vi "Pressure Write Array.vi"(8 "error in":errorcluster, 10 "Pressure AV":dbl[](array[numeric]), 11 "Chiller in":refnum<class "Chiller.lvclass">) -> (0 "error out":errorcluster, 3 "Chiller out":refnum<class "Chiller.lvclass">)   [LabVIEW 2023, in "Chiller.lvclass"]
uses:
  Chiller.lvclass
  Chiller.lvclass/Chiller.ctl
  Low Level Capabilities/Pressure/Pressure Actual Value/Pressure Actual Value.lvclass
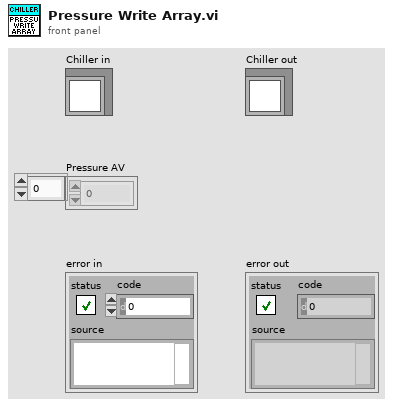
[diagram p1: front panel]
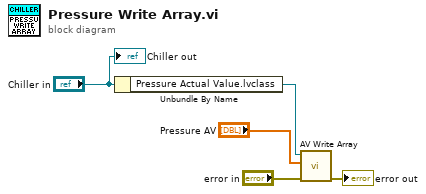
[diagram p0: block diagram]
diagram:
  n1 = Unbundle By Name("Chiller in") -> ("Pressure Actual Value.lvclass"=w5:refnum<class "Pressure Actual Value.lvclass">)
  n2 = call-dynamic "AV Write Array.vi"("error in"="error in", "Humidity AV"="Pressure AV", "Pressure Actual Value in"=w5) -> ("error out"=→"error out":errorcluster)  [unwired: 7 in, 1 out]
  "Chiller out" <- "Chiller in"
